vi "fill half sphere.vi"(0 "pict in":picture, 1 "size":i32(slide)=40 scale=0.0..50.0, 3 "v-matrix":dbl[][](array[numeric])=[[1.0, -0.0, 0.0, 0.0], [0.0, 1.0, 0.0, 0.0], [0.0, 0.0, 1.0, 0.0], [0.0, 0.0, 0.0, 1.0]], 4 "color gound":u32(colorbox)=52736, 5 "center":cluster{"x":i32, "y":i32}={"x"=51, "y"=51}, 8 "color sky":u32(colorbox)=10790143) -> (6 "pict out":picture)   [LabVIEW 2017]
uses:
  <vilib>/Analysis/baseanly.llb/Real A x B.vi
  <vilib>/Analysis/NI_AALBase.lvlib
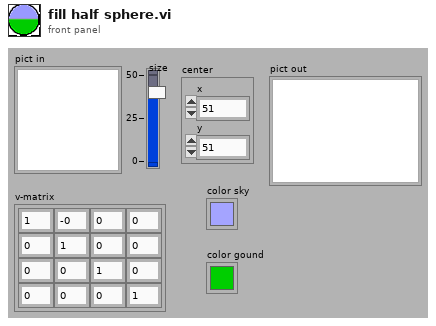
[diagram p1: front panel]
types:
  T1 = typedef "NI_Matrix.lvlib/RealMatrix.ctl" = dbl[][]
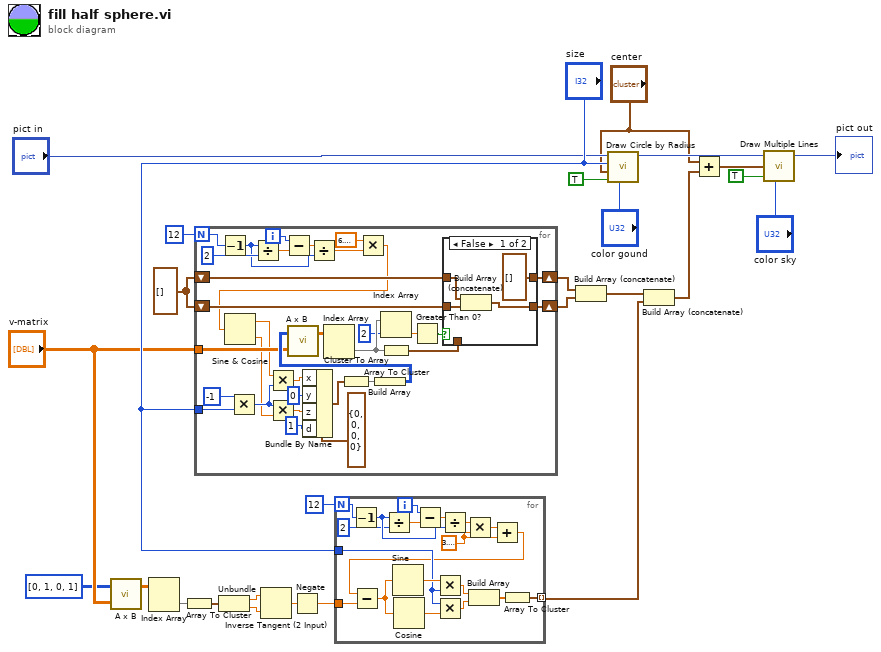
[diagram p0: block diagram]
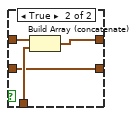
[diagram p2: hidden frame]
diagram:
  w21 = cluster{"A x B[0]":dbl, "A x B[1]":dbl}[] []
  n1 = call-poly <vilib>:"A x B.vi"("B"="v-matrix", "A"=i32[][] [[0, 1, 0, 1]]) -> ("A x B"=w25:T1)  [unwired: 1 out]
  n2 = Index Array(array=w25) -> (element=w13:dbl[])  [unwired: 2 in]
  n3 = Array To Cluster(array=w13) -> (cluster=w24:cluster{"A x B[0]":dbl, "A x B[1]":dbl})
  n4 = for {
    N: 12 ("y 2") -> [w55]
    tunnel: "size" -> [w43]
    shift-right: [w50] -> w22
    shift-left: w21 -> [w49]
    tunnel: "v-matrix" -> [w39]
    shift-right: [w33] -> w23
    shift-left: w21 -> [w32]
    i -> [w34]
    n5 = Decrement(x=w55) -> (x-1=w51:i32)
    n6 = Multiply(x=-1, y=w43) -> (x*y=w52:i32)
    n7 = Divide(x=w51, y=2) -> (x/y=w57:dbl)
    n8 = Subtract(x=w34, y=w57) -> (x-y=w53:dbl)
    n9 = Divide(x=w53, y=w51) -> (x/y=w42:dbl)
    n10 = Multiply(x=6.283185307179586, y=w42) -> (x*y=w30:dbl)
    n11 = Sine & Cosine(0:w30) -> (1:w29:dbl, 2:w28:dbl)
    n12 = Multiply(x=w29, y=w52) -> (x*y=w54:dbl)
    n13 = Multiply(x=w52, y=w28) -> (x*y=w38:dbl)
    n14 = Bundle By Name(cluster=cluster{"x":i16, "y":i16, "z":i16, "d":i16} {"x"=0, "y"=0, "z"=0, "d"=0}, "x"=w54, "y"=i16 0, "z"=w38, "d"=i16 1) -> (w60:cluster{"x":i16, "y":i16, "z":i16, "d":i16})
    n15 = Cluster To Array(cluster=w60) -> (array=w59:i16[])
    n16 = Build Array(w59) -> (w41:i16[][])
    n17 = call-poly <vilib>:"A x B.vi"("B"=w39, "A"=w41) -> ("A x B"=w40:T1)  [unwired: 1 out]
    n18 = Index Array(array=w40) -> (element=w48:dbl[])  [unwired: 2 in]
    n19 = Index Array(array=w48, index=2) -> (element=w47:dbl)
    n20 = Array To Cluster(array=w48) -> (cluster=w31:cluster{"A x B[0]":dbl, "A x B[1]":dbl})
    n21 = Greater Than 0?(x=w47) -> (x > 0?=w46:bool)
    n22 = case "Hide lines" shown="False" w46 {
      tunnel: [cluster{"A x B[0]":dbl, "A x B[1]":dbl}[] [] w68] -> w50
      tunnel: w49 -> [w61 w67]
      tunnel: w31 -> [_ w66]
      tunnel: [w63 w65] -> w33
      tunnel: w32 -> [w62 w65]
      frame False {
        n23 = Build Array (concatenate)(w61, w62) -> (w63:cluster{"A x B[0]":dbl, "A x B[1]":dbl}[])
      }
      frame True {
        n24 = Build Array (concatenate)(w67, w66) -> (w68:cluster{"A x B[0]":dbl, "A x B[1]":dbl}[])
      }
    }
  }
  n25 = Unbundle(w24) -> ("A x B[0]"=w15:dbl, "A x B[1]"=w11:dbl)
  n26 = Inverse Tangent (2 Input)(1:w11, 2:w15) -> (0:w16:dbl)
  n27 = Negate(x=w16) -> (-x=w12:dbl)
  n28 = for {
    N: 12 ("y 2") -> [w83]
    tunnel: "size" -> [w72]
    tunnel: [w71] -> w1 mode=indexing
    tunnel: w12 -> [w70]
    i -> [w82]
    w74 = 3.141592653589793
    n29 = Decrement(x=w83) -> (x-1=w87:i32)
    n30 = Divide(x=w87, y=2) -> (x/y=w84:dbl)
    n31 = Subtract(x=w82, y=w84) -> (x-y=w86:dbl)
    n32 = Divide(x=w86, y=w87) -> (x/y=w76:dbl)
    n33 = Multiply(x=w76, y=w74) -> (x*y=w75:dbl)
    n34 = Add(x=w75, y=w74) -> (x+y=w69:dbl)
    n35 = Subtract(x=w69, y=w70) -> (x-y=w80:dbl)
    n36 = Sine(x=w80) -> (sin(x)=w73:dbl)
    n37 = Cosine(x=w80) -> (cos(x)=w81:dbl)
    n38 = Multiply(x=w73, y=w72) -> (x*y=w78:dbl)
    n39 = Multiply(x=w72, y=w81) -> (x*y=w79:dbl)
    n40 = Build Array(w78, w79) -> (w77:dbl[])
    n41 = Array To Cluster(array=w77) -> (cluster=w71:cluster{"[0]":dbl, "[1]":dbl})
  }
  n42 = Build Array (concatenate)(w22, w23) -> (w19:cluster{"A x B[0]":dbl, "A x B[1]":dbl}[])
  n43 = call <vilib>:"Draw Circle by Radius.vi"("color(black)"="color gound", "fill?(F)"=TRUE, "pixel center"="center", "radius"="size", "picture"="pict in") -> ("new picture"=w18:picture)  [unwired: 6 in]
  n44 = Build Array (concatenate)(w19, w1) -> (w2:cluster{"[0]":dbl, "[1]":dbl}[])
  n45 = Add(x="center", y=w2) -> (x+y=w20:cluster{dbl, dbl}[])
  n46 = call <vilib>:"Draw Multiple Lines.vi"("picture"=w18, "line endpoints"=w20, "fill?(F)"=TRUE, "color(black)"="color sky") -> ("new picture"=→"pict out":picture)  [unwired: 5 in]
